vi "FGV_DOCK_REPORT_status_display.vi"(4 "front_panel_reference":refnum<vi>, 6 "status_display_reference":refnum<vi>, 7 "options":T1, 8 "error_in":errorcluster, 10 "SQL_statement":string, 11 "display_source":string) -> (0 "error_out":errorcluster)   [LabVIEW 2019]
uses:
  FGV_DOCK_REPORT_status_display.ctl
  _misc/AULocalize/SubVIs/Get Localized Phrase Compact Interface 0D.vi
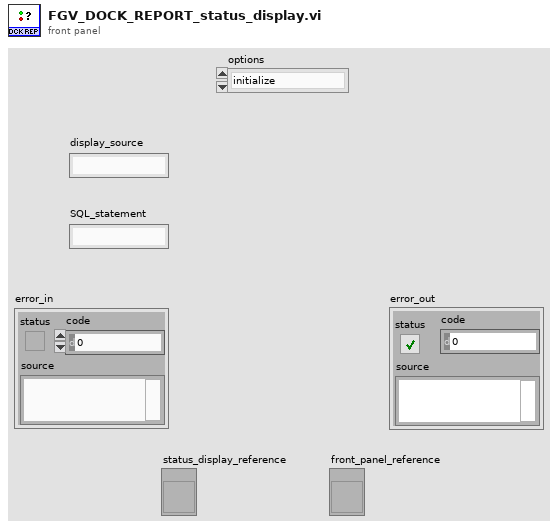
[diagram p1: front panel]
types:
  T1 = typedef "FGV_DOCK_REPORT_status_display.ctl" = enum16{"initialize", "display", "clear"}
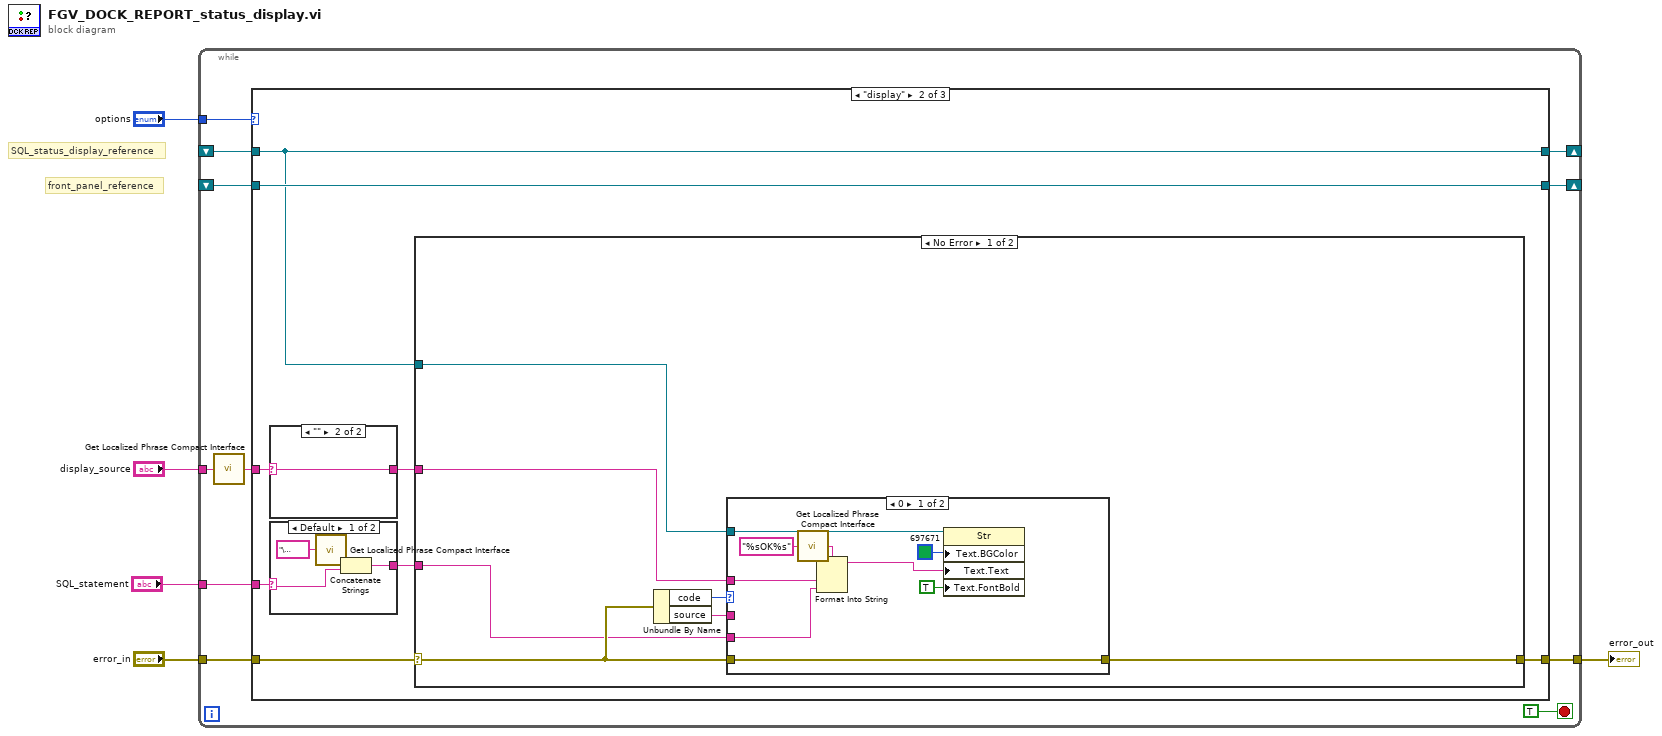
[diagram p0: block diagram]
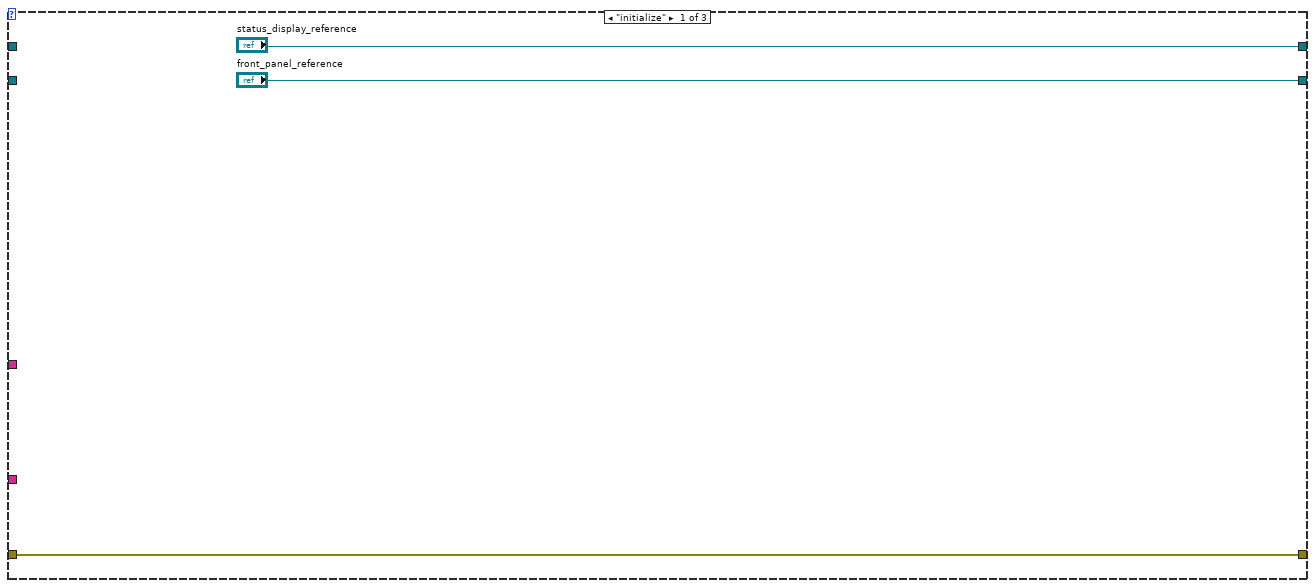
[diagram p2: hidden frame]
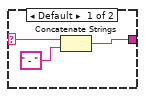
[diagram p4: hidden frame]
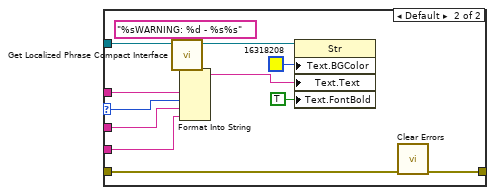
[diagram p5: hidden frame]
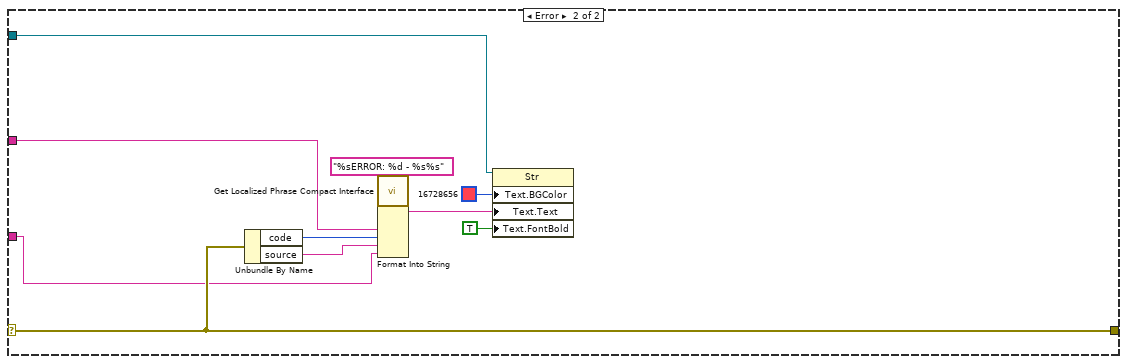
[diagram p6: hidden frame]
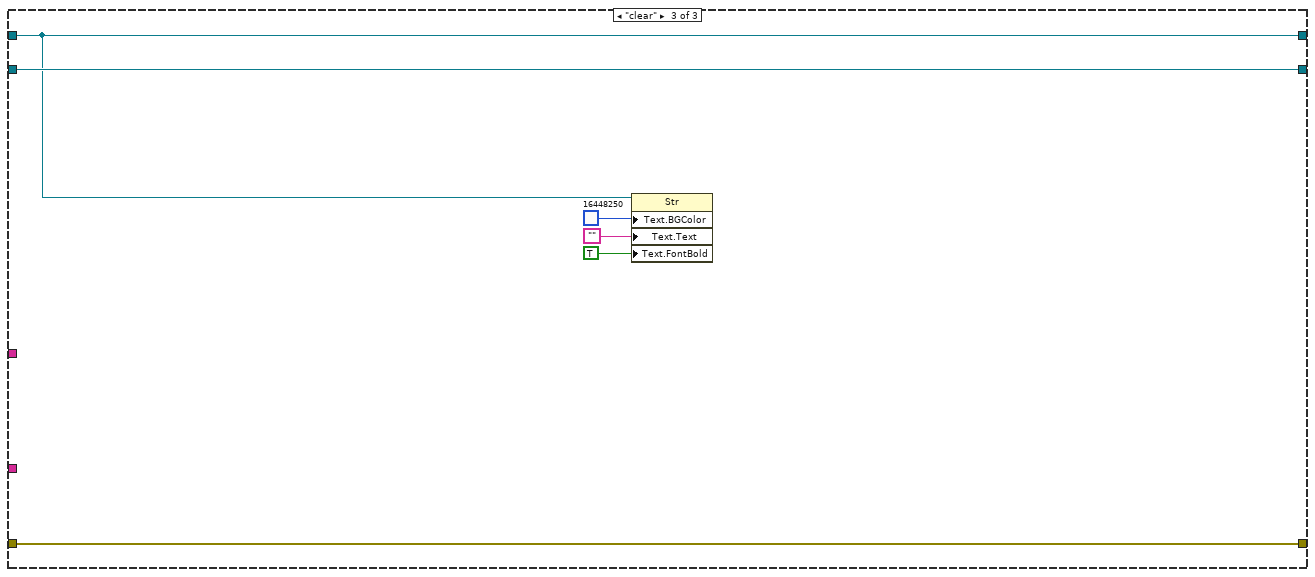
[diagram p7: hidden frame]
diagram:
  # "front_panel_reference"
  # "SQL_status_display_reference"
  n1 = while {
    tunnel: "options" -> [w15]
    tunnel: [w14] -> w5
    tunnel: "error_in" -> [w13]
    shift-right: [w12] -> _
    shift-left: _ -> [w11]
    shift-right: [w10] -> _
    shift-left: _ -> [w9]
    tunnel: "display_source" -> [w8]
    tunnel: "SQL_statement" -> [w7]
    stop <- TRUE stop-if-true
    n2 = call-poly "Get Localized Phrase Compact Interface.vi"("Key"=w8) -> ("Translated Phrase"=w6:string)
    n3 = case shown="\"display\"" w15 {
      tunnel: [w19 w26 w81] -> w14
      tunnel: w13 -> [w19 w27 w81]
      tunnel: ["status_display_reference" w24 w77] -> w12
      tunnel: w11 -> [_ w24 w77]
      tunnel: ["front_panel_reference" w25 w80] -> w10
      tunnel: w9 -> [_ w25 w80]
      tunnel: w6 -> [_ w23 _]
      tunnel: w7 -> [_ w21 _]
      frame "initialize" {
      }
      frame "display" {
        n4 = case shown="\"\"" w23 {
          selector: w23 -> [w35 w36]
          tunnel: [w34 w36] -> w22
          frame Default {
            n5 = Concatenate Strings(w35, " - " ("string")) -> (w34:string)
          }
          frame "" {
          }
        }
        n6 = case shown="Default" w21 {
          selector: w21 -> [w30 w32]
          tunnel: [w31 w32] -> w20
          frame Default {
            n7 = call-poly "Get Localized Phrase Compact Interface.vi"("Key"="\nExecuted SQL statement: " ("string")) -> ("Translated Phrase"=w28:string)
            n8 = Concatenate Strings(w28, w30) -> (w31:string)
          }
          frame "" {
          }
        }
        n9 = case shown="No Error" w27 {
          selector: w27 -> [w40 w69]
          tunnel: [w39 w69] -> w26
          tunnel: w24 -> [w42 w68]
          tunnel: w22 -> [w38 w67]
          tunnel: w20 -> [w37 w66]
          frame No Error {
            n10 = Unbundle By Name(w40) -> ("code"=w41:i32, "source"=w43:string)
            n11 = case shown="0" w41 {
              selector: w41 -> [_ w58]
              tunnel: w43 -> [_ w63]
              tunnel: w42 -> [w50 w59]
              tunnel: w40 -> [w49 w56]
              tunnel: [w49 w57] -> w39
              tunnel: w38 -> [w47 w55]
              tunnel: w37 -> [w45 w54]
              frame 0 {
                n12 = call-poly "Get Localized Phrase Compact Interface.vi"("Key"="%sOK%s" ("Text.Text")) -> ("Translated Phrase"=w44:string)
                n13 = Format Into String(format string=w44, w47, w45) -> (resulting string=w46:string)  [unwired: 2 in, 1 out]
                n14 = property on="Property Node" class="Str"(reference=w50, "Text.BGColor"=u32 697671, "Text.Text"=w46, "Text.FontBold"=TRUE ("Text.Font:Bold")) -> ()  [unwired: 1 in, 2 out]
              }
              frame Default {
                n15 = call-poly "Get Localized Phrase Compact Interface.vi"("Key"="%sWARNING: %d - %s%s" ("format string")) -> ("Translated Phrase"=w53:string)
                n16 = Format Into String(format string=w53, w55, w58, w63, w54) -> (resulting string=w62:string)  [unwired: 2 in, 1 out]
                n17 = property on="Property Node" class="Str"(reference=w59, "Text.BGColor"=u32 16318208, "Text.Text"=w62, "Text.FontBold"=TRUE ("Text.Font:Bold")) -> ()  [unwired: 1 in, 2 out]
                n18 = call <vilib>:"Clear Errors.vi"("error in (no error)"=w56) -> ("error out"=w57:errorcluster)  [unwired: 5 in, 1 out]
              }
            }
          }
          frame Error {
            n19 = Unbundle By Name(w69) -> ("code"=w74:i32, "source"=w73:string)
            n20 = call-poly "Get Localized Phrase Compact Interface.vi"("Key"="%sERROR: %d - %s%s" ("format string")) -> ("Translated Phrase"=w65:string)
            n21 = Format Into String(format string=w65, w67, w74, w73, w66) -> (resulting string=w72:string)  [unwired: 2 in, 1 out]
            n22 = property on="Property Node" class="Str"(reference=w68, "Text.BGColor"=u32 16728656 ("Color Box"), "Text.Text"=w72, "Text.FontBold"=TRUE ("Text.Font:Bold")) -> ()  [unwired: 1 in, 2 out]
          }
        }
      }
      frame "clear" {
        n23 = property on="Property Node" class="Str"(reference=w77, "Text.BGColor"=u32 16448250, "Text.Text"="", "Text.FontBold"=TRUE ("Text.Font:Bold")) -> ()  [unwired: 1 in, 2 out]
      }
    }
  }
  "error_out" <- w5
